vi "_script_rel_path.vi"(10 "Child":path, 11 "Parent":path) -> (3 "Child Relative Path":path)   [LabVIEW 2019, in "Script.lvlib"]
doc: "Returns the relative path of the child path to the parent path.\n\nCreated by: Ryan Pacini"
uses:
  Script.lvlib
panel:
  out "Common Path":path
  out "Child Relative to Parent":bool
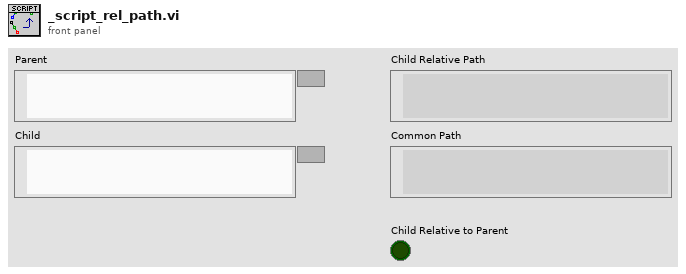
[diagram p1: front panel]
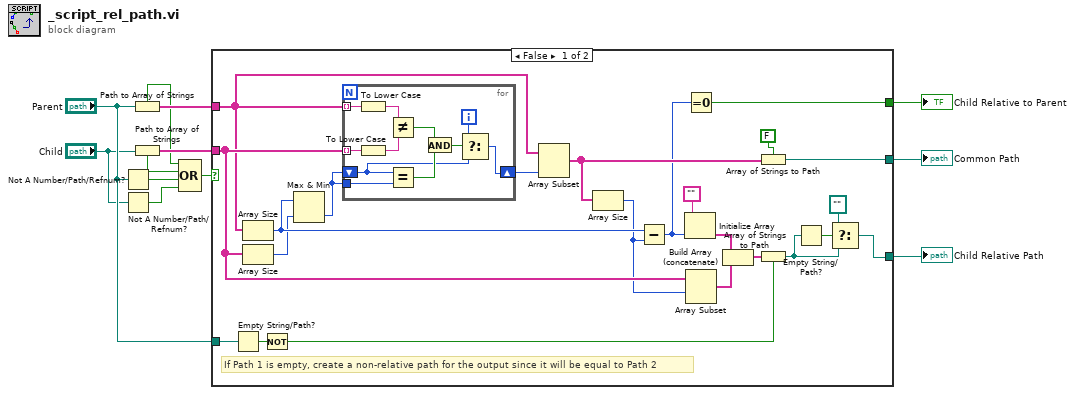
[diagram p0: block diagram]
diagram:
  n1 = Not A Number/Path/Refnum?(number/path/refnum="Parent") -> (NaN/Path/Refnum?=w2:bool)
  n2 = Not A Number/Path/Refnum?(number/path/refnum="Child") -> (NaN/Path/Refnum?=w1:bool)
  n3 = Path to Array of Strings(0:"Parent") -> (1:w3:bool, 2:w7:string[])
  n4 = Path to Array of Strings(0:"Child") -> (1:w4:bool, 2:w6:string[])
  n5 = Compound Arithmetic op=OR(w3, w4, w2, w1) -> (w5:bool)
  n6 = case shown="False" w5 {
    tunnel: w7 -> [w27 _]
    tunnel: w6 -> [w30 _]
    tunnel: [w33 _] -> w10
    tunnel: [w14 _] -> w9
    tunnel: [w21 _] -> w8
    tunnel: "Parent" -> [w19 _]
    frame False {
      # "If Path 1 is empty, create a non-relative path for the output since it will be equal to Path 2"
      n7 = Empty String/Path?(string/path=w19) -> (empty?=w18:bool)
      n8 = Array Size(array=w27) -> (size(s)=w26:i32)
      n9 = Array Size(array=w30) -> (size(s)=w25:i32)
      n10 = Not(x=w18) -> (.not. x?=w17:bool)
      n11 = Max & Min(x=w26, y=w25) -> (min(x,y)=w24:i32)  [unwired: 1 out]
      n12 = for {
        tunnel: w27 -> [w46] mode=indexing
        tunnel: w30 -> [w45] mode=indexing
        shift-right: [w38] -> w35
        shift-left: w24 -> [w39]
        tunnel: w24 -> [w44]
        i -> [w40]
        n13 = To Lower Case(string=w46) -> (all lower case string=w37:string)
        n14 = To Lower Case(string=w45) -> (all lower case string=w36:string)
        n15 = Not Equal?(x=w37, y=w36) -> (x != y?=w42:bool)
        n16 = Equal?(x=w39, y=w44) -> (x = y?=w43:bool)
        n17 = And(x=w42, y=w43) -> (x .and. y?=w41:bool)
        n18 = Select(t=w40, s=w41, f=w39) -> (s? t:f=w38:i32)
      }
      n19 = Array Subset(array=w27, length=w35) -> (w32:string[])  [unwired: 1 in]
      n20 = Array Size(array=w32) -> (size(s)=w23:i32)
      n21 = Subtract(x=w26, y=w23) -> (x-y=w22:i32)
      n22 = Initialize Array("", w22) -> (w31:string[])
      n23 = Equal To 0?(x=w22) -> (x = 0?=w21:bool)
      n24 = Array Subset(array=w30, index=w23) -> (w29:string[])  [unwired: 1 in]
      n25 = Build Array (concatenate)(w31, w29) -> (w28:string[])
      n26 = Array of Strings to Path(0:w32, 1:FALSE ("relative")) -> (2:w33:path)
      n27 = Array of Strings to Path(0:w28, 1:w17) -> (2:w15:path)
      n28 = Empty String/Path?(string/path=w15) -> (empty?=w16:bool)
      n29 = Select(t=path "", s=w16, f=w15) -> (s? t:f=w14:path)
    }
    frame True {
      # "If either of the paths are relative, or not a path, return error 1430."
    }
  }
  "Child Relative Path" <- w9
  "Child Relative to Parent" <- w8
  "Common Path" <- w10
